vi "instance count allowed.vi"(8 "error in":errorcluster, 11 "configuration in":refnum<class "TBM module configuration.lvclass">) -> (0 "error out":errorcluster, 2 "instances allowed":i32, 3 "configuration out":refnum<class "TBM module configuration.lvclass">)   [LabVIEW 2013, in "TBM module configuration.lvclass"]
doc: "Provides an interface for determining the reentrancy of the runtime class associated with this configuration class. For example, a module which performs processing tasks may allow for unlimited instances (-1) while a component which implements a TCP server may want to limit itself to a smaller number in order to preserve ports. configuration.lvclass provides a value of 0, as no runtime class exists for this configuration.Copyright 2015 National Instruments Corporation\n\nLicensed under the Apache License, Version 2.0 (the \"License\"); you may not use this file except in compliance with the License. You may obtain a copy of the License at http://www.apache.org/licenses/LICENSE-2.0\nUnless required by applicable law or agreed to in writing, software distributed under the License is distributed on an \"AS IS\" BASIS, WITHOUT WARRANTIES OR CONDITIONS OF ANY KIND, either express or implied. See the License for the specific language governing permissions and limitations under the License."
uses:
  TBM module configuration.lvclass
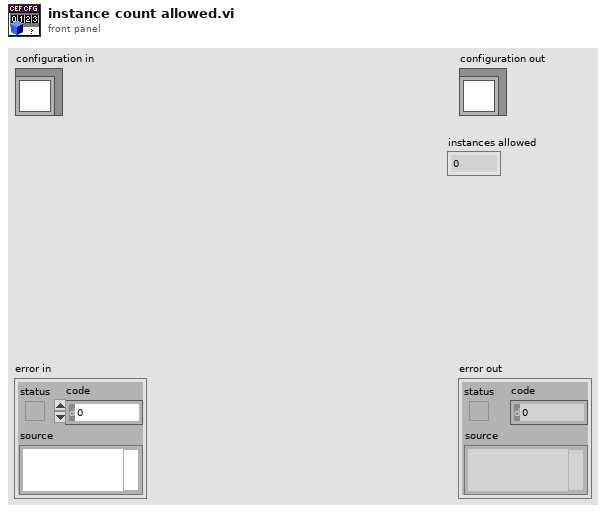
[diagram p1: front panel]
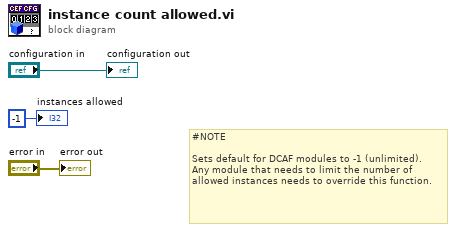
[diagram p0: block diagram]
diagram:
  # "#NOTE\n\nSets default for DCAF modules to -1 (unlimited).\nAny module that needs to limit the number of allowed instances needs to override this function."
  "error out" <- "error in"
  "configuration out" <- "configuration in"
  "instances allowed" <- -1 ("instances allowed")
